vi "GetSubPanelVIName.vi"(0 "VIName":string, 5 "SubPanelLabel":string="Sub Panel", 11 "error in (no error)":errorcluster) -> (4 "VI Name":string, 15 "error out":errorcluster)   [LabVIEW 2021]
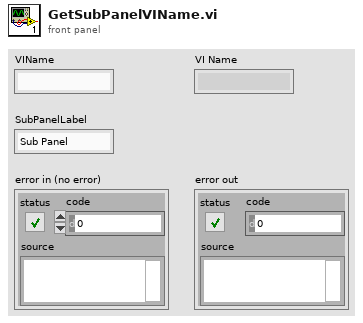
[diagram p1: front panel]
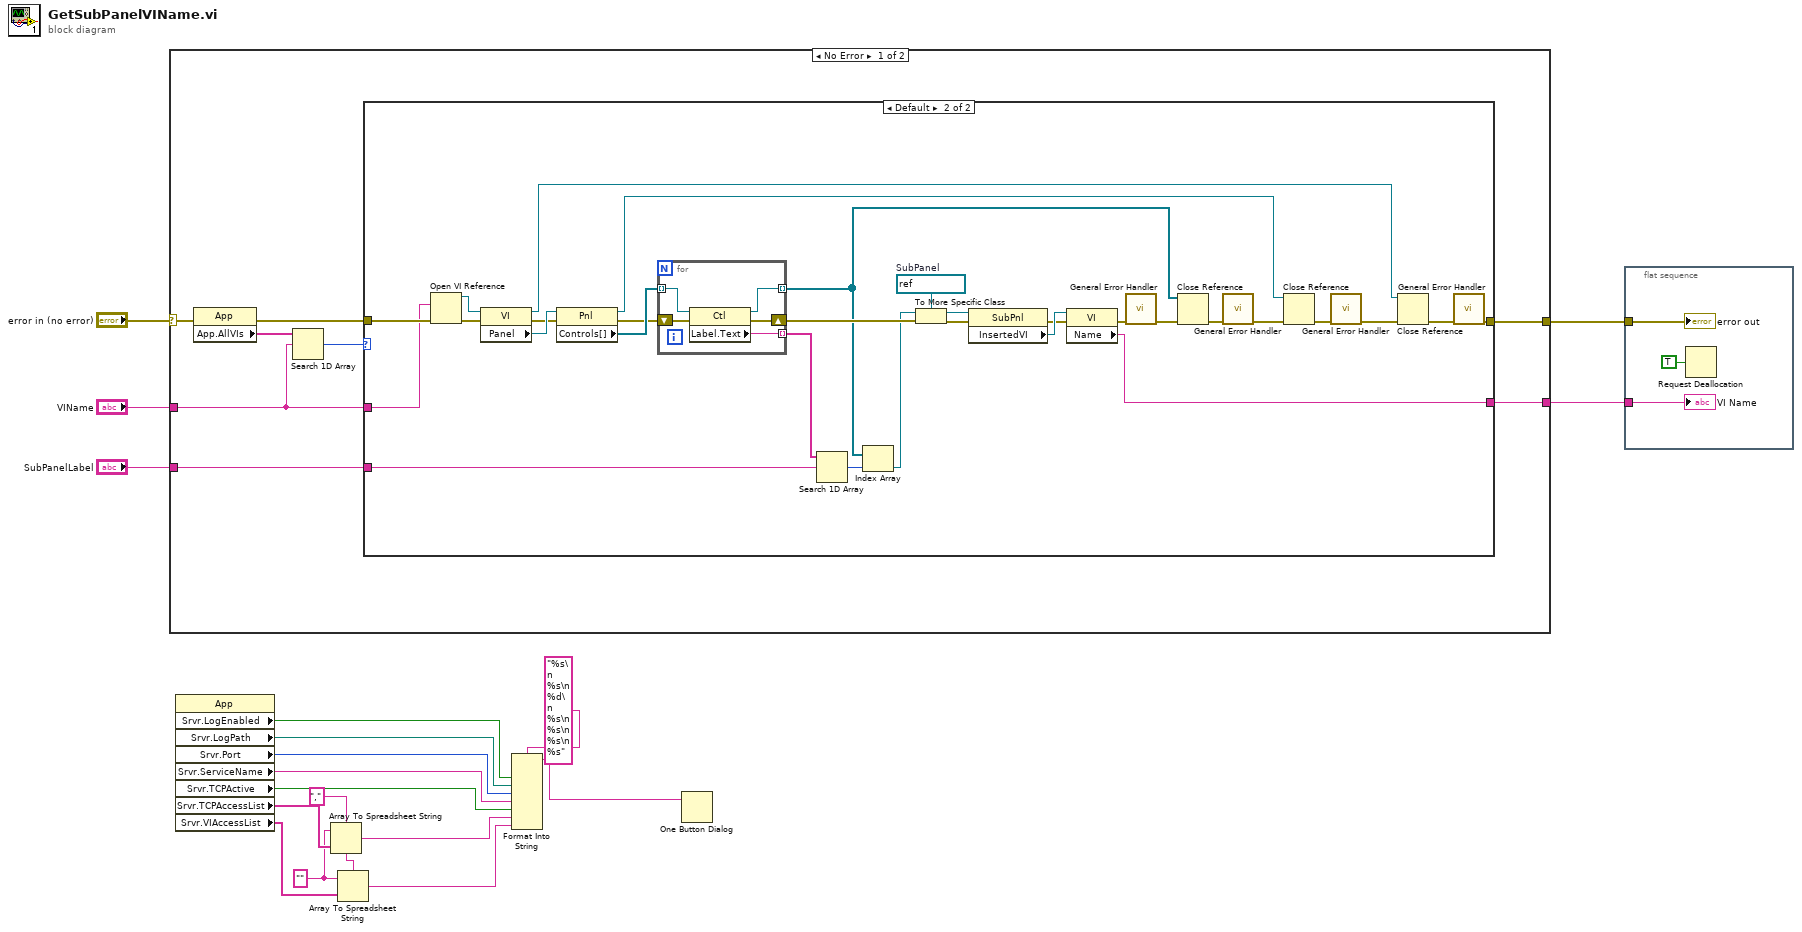
[diagram p0: block diagram]
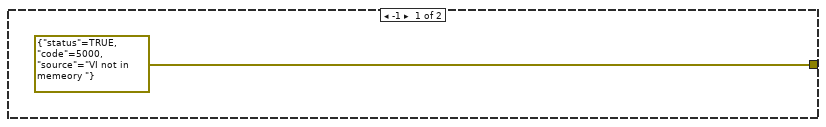
[diagram p2: hidden frame]
diagram:
  w1 = "" ("format string")
  w6 = "," ("delimiter (Tab)")
  n1 = case shown="No Error" "error in (no error)" {
    selector: "error in (no error)" -> [w26 w63]
    tunnel: "VIName" -> [w20 _]
    tunnel: [w25 w63] -> w16
    tunnel: "SubPanelLabel" -> [w24 _]
    tunnel: [w23 _] -> w14
    frame No Error {
      n2 = property class="App"(error in=w26) -> (error out=w22:errorcluster, "App.AllVIs"=w21:string[])  [unwired: 1 in, 1 out]
      n3 = Search 1D Array(1D array=w21, element=w20) -> (index of element=w19:i32)  [unwired: 1 in]
      n4 = case shown="Default" w19 {
        tunnel: [errorcluster {"status"=TRUE, "code"=5000, "source"="VI not in memeory "} ("error out") w28] -> w25
        tunnel: w24 -> [_ w41]
        tunnel: [_ w37] -> w23
        tunnel: w22 -> [_ w35]
        tunnel: w20 -> [_ w34]
        frame -1 {
        }
        frame Default {
          w56 = refnum<vi> refnum  # SubPanel
          n5 = Open VI Reference(vi path=w34, error in (no error)=w35) -> (vi reference=w52:refnum<vi>, error out=w51:errorcluster)  [unwired: 4 in]
          n6 = property class="VI"(reference=w52, error in=w51) -> (reference out=w44:refnum<vi>, error out=w50:errorcluster, "Panel"=w53:refnum<vi>)
          n7 = property class="Pnl"(reference=w53, error in=w50) -> (reference out=w43:refnum<vi>, error out=w49:errorcluster, "Controls[]"=w54:refnum<vi>[])
          n8 = for {
            tunnel: w54 -> [w62] mode=indexing
            tunnel: [w61] -> w42 mode=indexing
            shift-right: [w58] -> w48
            shift-left: w49 -> [w59]
            tunnel: [w60] -> w38 mode=indexing
            n9 = property class="Ctl"(reference=w62, error in=w59) -> (reference out=w60:refnum<vi>, error out=w58:errorcluster, "Label.Text"=w61:string)
          }
          n10 = Search 1D Array(1D array=w42, element=w41) -> (index of element=w40:i32)  [unwired: 1 in]
          n11 = Index Array(array=w38, index=w40) -> (element=w39:refnum<vi>)
          n12 = To More Specific Class(target class=w56, reference=w39, error in=w48) -> (specific class reference=w55:refnum<vi>, error out=w47:errorcluster)
          n13 = property class="SubPnl"(reference=w55, error in=w47) -> (error out=w46:errorcluster, "InsertedVI"=w57:refnum<vi>)  [unwired: 1 out]
          n14 = property class="VI"(reference=w57, error in=w46) -> (error out=w36:errorcluster, "Name"=w37:string)  [unwired: 1 out]
          n15 = call <vilib>:"General Error Handler.vi"("error in (no error)"=w36) -> ("error out"=w31:errorcluster)  [unwired: 10 in, 4 out]
          n16 = Close Reference(reference=w38, error in (no error)=w31) -> (error out=w32:errorcluster)
          n17 = call <vilib>:"General Error Handler.vi"("error in (no error)"=w32) -> ("error out"=w30:errorcluster)  [unwired: 10 in, 4 out]
          n18 = Close Reference(reference=w43, error in (no error)=w30) -> (error out=w33:errorcluster)
          n19 = call <vilib>:"General Error Handler.vi"("error in (no error)"=w33) -> ("error out"=w29:errorcluster)  [unwired: 10 in, 4 out]
          n20 = Close Reference(reference=w44, error in (no error)=w29) -> (error out=w45:errorcluster)
          n21 = call <vilib>:"General Error Handler.vi"("error in (no error)"=w45) -> ("error out"=w28:errorcluster)  [unwired: 10 in, 4 out]
        }
      }
    }
    frame Error {
    }
  }
  n22 = property class="App"() -> ("Srvr.LogEnabled"=w13:bool, "Srvr.LogPath"=w12:path, "Srvr.Port"=w11:u32, "Srvr.ServiceName"=w10:string, "Srvr.TCPActive"=w9:bool, "Srvr.TCPAccessList"=w8:string[], "Srvr.VIAccessList"=w7:string[])  [unwired: 2 in, 2 out]
  n23 = Array To Spreadsheet String(delimiter (Tab)=w6, array=w8, 3:w1) -> (spreadsheet string=w5:string)
  n24 = Array To Spreadsheet String(delimiter (Tab)=w6, array=w7, 3:w1) -> (spreadsheet string=w4:string)
  n25 = Format Into String(format string="%s\n %s\n %d\n %s\n %s\n %s\n %s", w13, w12, w11, w10, w9, w5, w4) -> (resulting string=w2:string)  [unwired: 2 in, 1 out]
  n26 = One Button Dialog(message=w2) -> ()  [unwired: 1 in, 1 out]
  n27 = flat-sequence {
    tunnel: w16 -> [w66]
    tunnel: w14 -> [w65]
    frame #0 {
      n28 = Request Deallocation(TRUE ("flag")) -> ()
      "error out" <- w66
      "VI Name" <- w65
    }
  }
